vi "STM Write Meta Data (UDP Clst).vi"(4 "Address":cluster{"address":u32, "port":u16}, 6 "Options":T3={"Ignore Timeout Error"=TRUE, "timeout ms (1000)"=1000}, 7 "Meta data":T2[](array[typedef]), 8 "error in":errorcluster, 11 "Connection Info In":T1) -> (0 "error out":errorcluster, 3 "Connection Info Out":T1)   [LabVIEW 2010]
doc: "Use this VI to transmit the meta data cluster to a remote computer. Sending the meta data to another computer helps maintainability since the data resides only on one side and it is shared to other computers at run time."
uses:
  stm_MetaDataElement.ctl
  stm_UDP Connection Info.ctl
  stm_UDP Write Options.ctl
  NI STM.lvlib
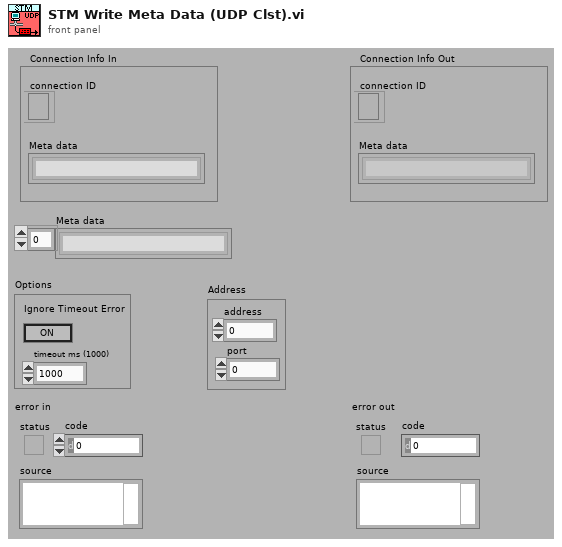
[diagram p1: front panel]
types:
  T1 = typedef "stm_UDP Connection Info.ctl" = cluster{"connection ID":refnum<k16>, "Meta data":T2[]}
  T2 = typedef "stm_MetaDataElement.ctl" = string
  T3 = typedef "stm_UDP Write Options.ctl" = cluster{"Ignore Timeout Error":bool, "timeout ms (1000)":i32}
  T4 = typedef "NI STM.lvlib/UDP Connection Info.ctl" = cluster{"connection ID":refnum<k16>, "Meta data":T5[]}
  T5 = typedef "NI STM.lvlib/MetaDataElement.ctl" = string
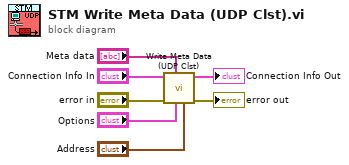
[diagram p0: block diagram]
diagram:
  n1 = call "Write Meta Data (UDP Clst).vi"("Address"="Address", "Options"="Options", "Meta data"="Meta data", "error in"="error in", "Connection Info In"="Connection Info In") -> ("error out"=→"error out":errorcluster, "Connection Info Out"=→"Connection Info Out":T4)  [unwired: 5 in]
